vi "NaN or null to Integer ERROR.vi"(8 "error in (no error)":errorcluster, 10 "JSON NaN or null":string) -> (0 "error out":errorcluster)   [LabVIEW 2017, in "JSONtext.lvlib"]
uses:
  JSONtext.lvlib
  <vilib>/Utility/error.llb/Error Cluster From Error Code.vi
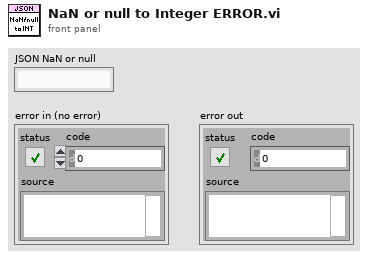
[diagram p1: front panel]
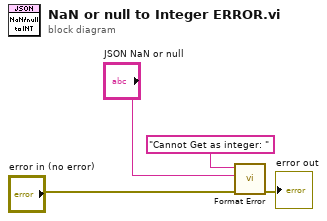
[diagram p0: block diagram]
diagram:
  n1 = call "Format Error.vi"("error in (no error)"="error in (no error)", "message part 2"="JSON NaN or null", "error message"="Cannot Get as integer: " ("format string")) -> ("error out"=→"error out":errorcluster)  [unwired: 8 in]
